vi "IFFT Bin interpolation.vi"(0 "Max Bin":i32, 1 "Max Amp":dbl, 2 "Prev Max Amp":dbl, 3 "Succ Max Amp":dbl, 4 "Windowing":T1(ring)) -> (5 "Interpolate Bin":dbl)   [LabVIEW 2014]
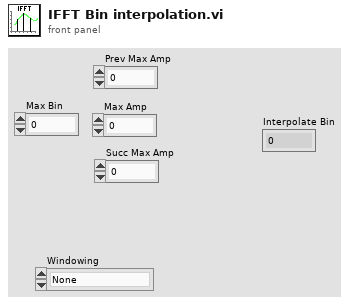
[diagram p1: front panel]
types:
  T1 = enum16{"None", "Hanning", "Hamming", "Blackman", "Blackman-Harris"}
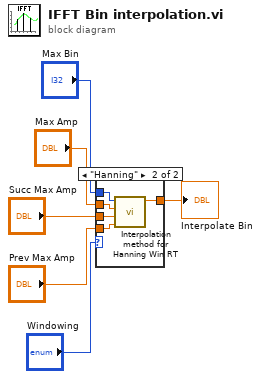
[diagram p0: block diagram]
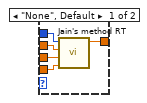
[diagram p2: hidden frame]
diagram:
  n1 = case shown="\"Hanning\"" "Windowing" {
    tunnel: [w11 w16] -> w1
    tunnel: "Max Bin" -> [w10 w15]
    tunnel: "Max Amp" -> [w9 w14]
    tunnel: "Succ Max Amp" -> [w8 w13]
    tunnel: "Prev Max Amp" -> [w7 w12]
    frame "None", Default {
      n2 = call "Jain's method RT.vi"("Prev Amp"=w7, "Next Amp"=w8, "Max Amp"=w9, "Max Bin"=w10) -> ("Bin"=w11:dbl)  [unwired: 7 in]
    }
    frame "Hanning" {
      n3 = call "Interpolation method for Hanning Win RT.vi"("Prev Amp"=w12, "Next Amp"=w13, "Max Amp"=w14, "Max Bin"=w15) -> ("Bin"=w16:dbl)  [unwired: 7 in]
    }
  }
  "Interpolate Bin" <- w1
